vi "Test Base Namer no extension no label.vi"   [LabVIEW 2020, in "Namer.Tests.lvclass"]
uses:
  Namer.Tests.lvclass
  Source/Approval Tests/Namer/Namer.lvclass
  Source/Approval Tests/Naming Data/Naming Data.lvclass
  Source/Approval Tests/Naming Data/Naming Data.lvclass/Naming Data.ctl
  <vilib>/addons/_JKI Toolkits/Caraya/classes/Test/Test.lvclass
  <vilib>/addons/_JKI Toolkits/Caraya/classes/Assert/Assert.lvclass
  <vilib>/addons/_JKI Toolkits/Caraya/classes/Assert/Assert Equal Value and Type_Variant.vi
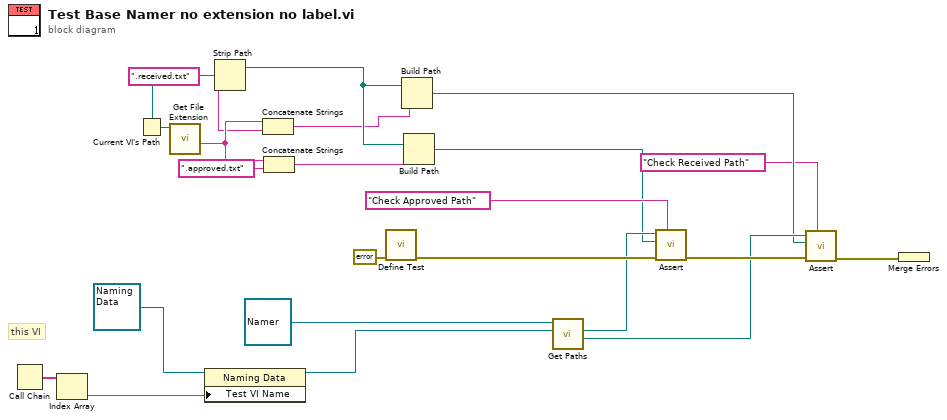
[diagram p0: block diagram]
diagram:
  # "this VI"
  n1 = Call Chain() -> (call chain=w17:string[])
  n2 = Index Array(array=w17) -> (element=w16:string)  [unwired: 1 in]
  n3 = Current VI's Path() -> (path=w10:path)
  n4 = call <vilib>:"Get File Extension.vi"("file"=w10) -> ("filename without extension"=w8:string)  [unwired: 6 in, 4 out]
  n5 = property on="Property Node" class="Naming Data"(reference=refnum<class "Naming Data.lvclass"> refnum ("Naming Data"), "Test VI Name"=w16) -> (reference out=w15:refnum<class "Naming Data.lvclass">)  [unwired: 1 in, 1 out]
  n6 = Strip Path(path=w10) -> (stripped path=w9:path)  [unwired: 1 out]
  n7 = Concatenate Strings(w8, ".received.txt" ("string")) -> (w5:string)
  n8 = Concatenate Strings(w8, ".approved.txt" ("string")) -> (w4:string)
  n9 = call <vilib>:"Define Test.vi"("error in (no error)"=errorcluster {"status"=FALSE, "code"=0, "source"=""}) -> ("error out"=w21:errorcluster)  [unwired: 9 in, 1 out]
  n10 = Build Path(base path=w9, name or relative path=w5) -> (appended path=w3:path)
  n11 = Build Path(base path=w9, name or relative path=w4) -> (appended path=w2:path)
  n12 = call-dynamic "Get Paths.vi"("Naming Data"=w15, "Namer in"=refnum<class "Namer.lvclass"> refnum ("Approval Tests:Namer")) -> ("Received Path"=w11:path, "Approved Path"=w12:path)  [unwired: 6 in, 2 out]
  n13 = call-poly <vilib>:"Assert.vi"("Label"="Check Approved Path" ("Label (VI Title)"), "error in (no error)"=w21, "Actual"=w2, "Expected"=w12) -> ("error out"=w14:errorcluster)  [unwired: 6 in, 1 out]
  n14 = call-poly <vilib>:"Assert.vi"("Label"="Check Received Path" ("Label (VI Title)"), "error in (no error)"=w14, "Actual"=w3, "Expected"=w11) -> ("error out"=w13:errorcluster)  [unwired: 6 in, 1 out]
  n15 = Merge Errors(w13) -> ()  [unwired: 1 out]
